vi "四图表串口字符转数字显示.vi"() -> ()   [LabVIEW 2013]
uses:
  <vilib>/Platform/TimedLoop/XDataNode/timing_clust.ctl
  <vilib>/Platform/TimedLoop/XDataNode/nitl_modes.ctl
  <vilib>/Platform/TimedLoop/XDataNode/wakeup.ctl
  <vilib>/Instr/_visa.llb/VISA Configure Serial Port (Instr).vi
  <vilib>/Platform/TimedLoop/XDataNode/XDataNode.xnode
  <vilib>/Platform/TimedLoop/XDataNode/XDNodeRunTimeDep.lvlib
panel:
  out "?":bool
  out "?":bool
  out "?":bool
  in  "预警低温 2":dbl=-5.0
  in  "预警高温 2":dbl=40.0
  out "?":bool
  in  "预警低温":dbl=-5.0
  in  "预警高温":dbl=40.0
  out "光照指示":bool
  in  "关灯时间":timestamp format="%<%H:%M:%S>T"
  in  "?":bool
  in  "?":bool
  out "LED灯":bool
  out "?":dbl
  out "湿度2":u8(graph)
  out "?":dbl
  out "温度2":u8(graph)
  in  "?":bool
  in  "?":bool
  out "?":dbl
  out "?":dbl
  out "红外指示灯":bool
  out "LED灯":bool
  out "湿度1":u8(graph)
  out "温度1":u8(graph)
  out "数值":u32
  in  "开始":bool
  in  "串口号":refnum<visa-resource-name>
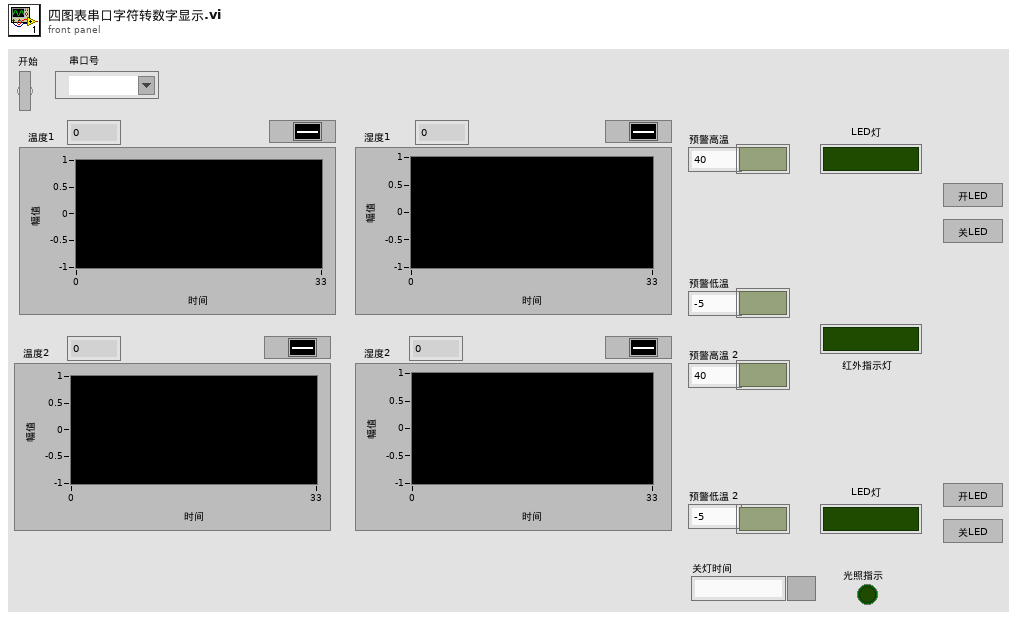
[diagram p1: front panel]
types:
  T1 = typedef "XDNodeRunTimeDep.lvlib/timing_clust.ctl" = cluster{"Expected End [f-1]":u64, "Actual End [f-1]":u64, "Finished Late? [f-1]":bool, "Expected End [i-1]":u64, "Actual End [i-1]":u64, "Finished Late? [i-1]":bool, "Expected Start [i]":u64, "Actual Start [i]":u64, "Expected Start [f]":u64, "Actual Start [f]":u64, "Source Name":string, "Structure Name":string, "Period":i64, "Deadline":i64, "Offset":i64, "Start":i64, "Priority":i32, "Timeout":i32, "Mode":T2, "Wakeup Reason":T3, "Error":errorcluster, "Source Type":string, "Secondary Source Type":string, "Global End Time":u64, "Global Start Time":u64, "Frame Duration":u64, "Iteration Duration":u64, "Assigned CPU":i32, "I/O Scan Engine Mode":u32}
  T2 = typedef "XDNodeRunTimeDep.lvlib/nitl_modes.ctl" = enum32{"No Change", "Process missed periods, maintain original phase", "Discard missed periods, maintain original phase", "Process missed periods, ignore original phase", "Discard missed periods, ignore original phase"}
  T3 = typedef "XDNodeRunTimeDep.lvlib/wakeup.ctl" = enum32{"Normal", "Aborted", "Asynchronous wakeup", "Timing source error", "Timed loop error", "Timeout"}
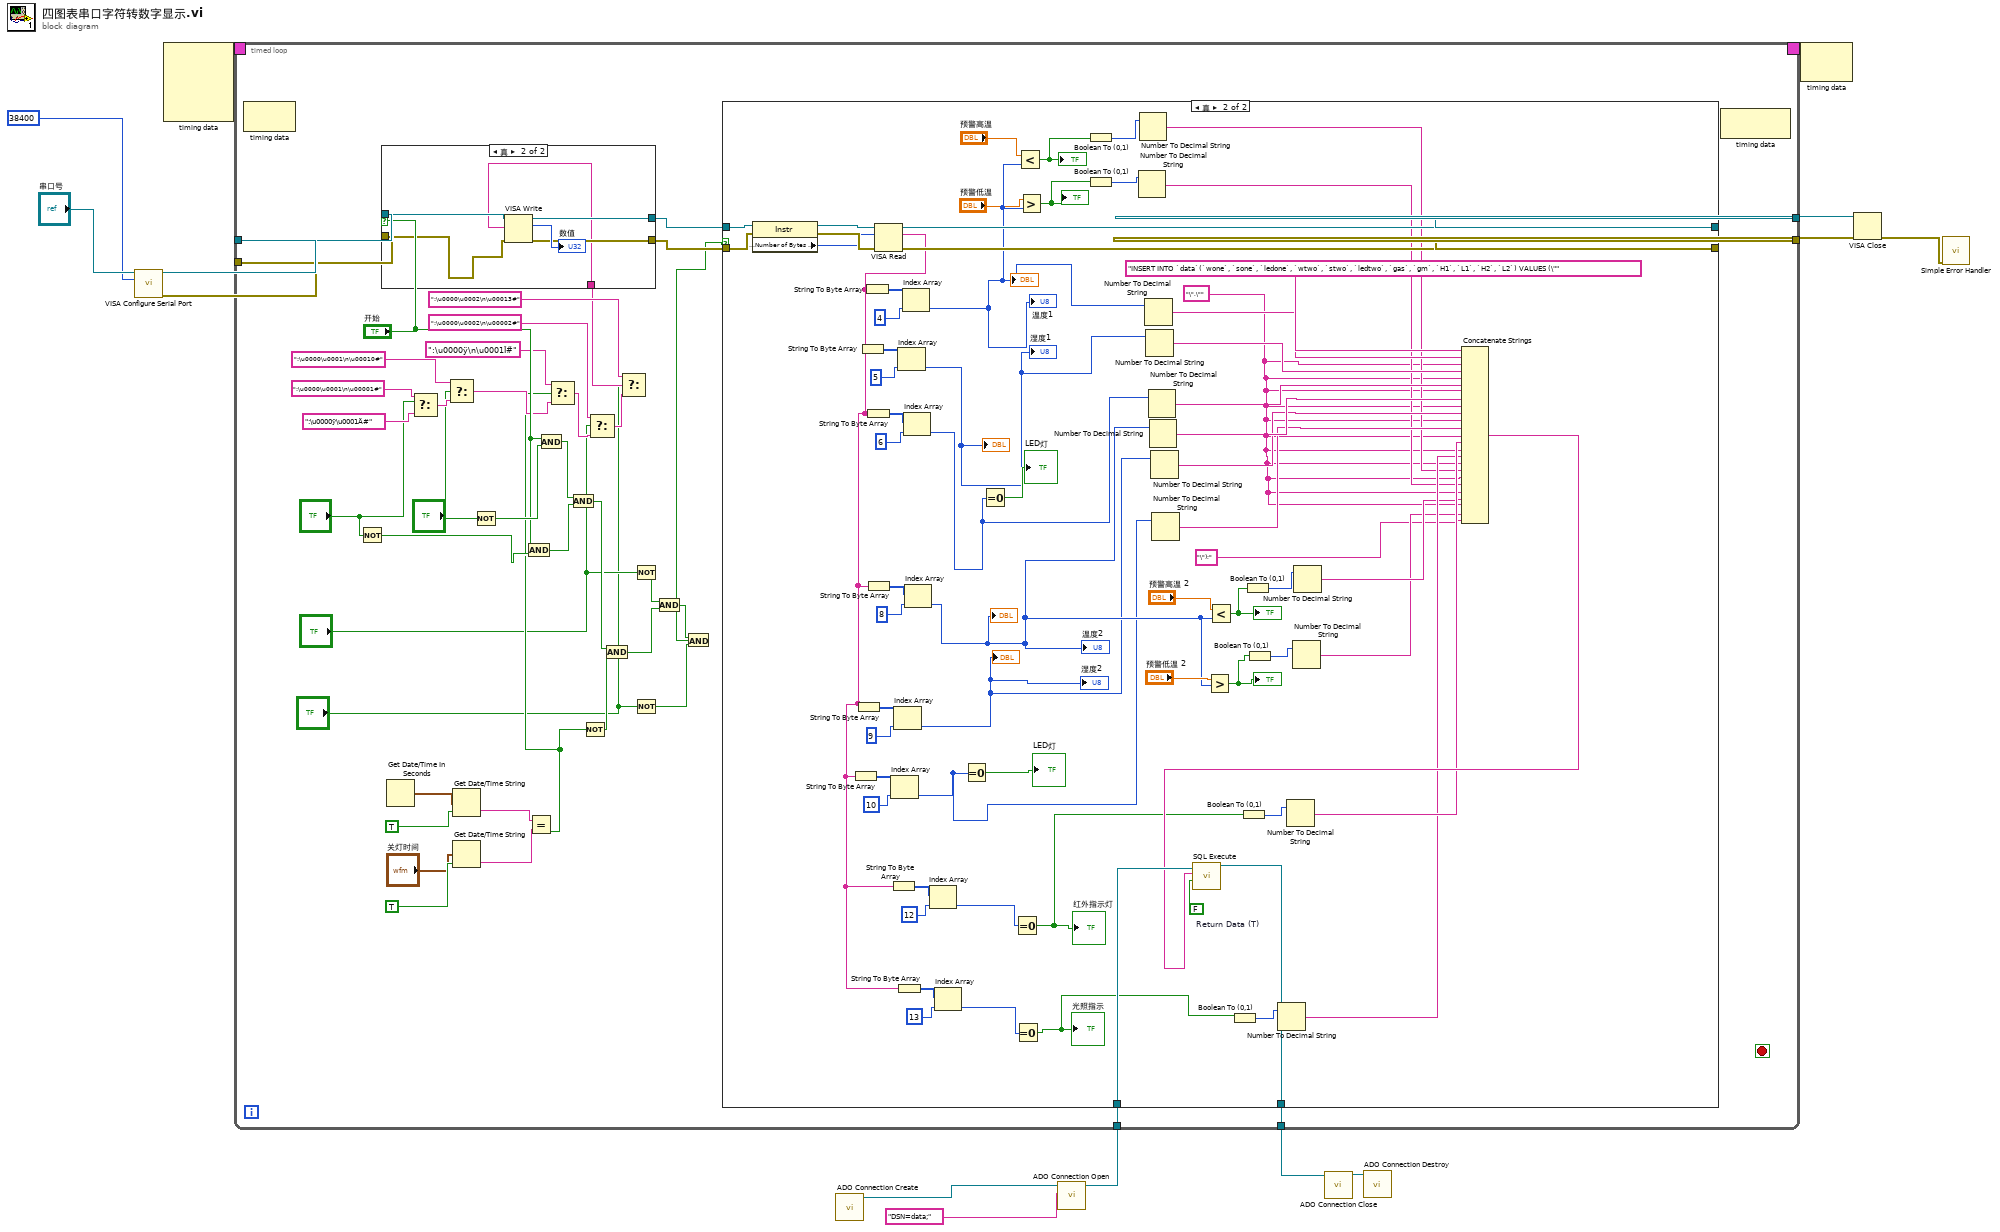
[diagram p0: block diagram]
diagram:
  n1 = call-poly "VISA Configure Serial Port"("VISA resource name"="串口号", "baud rate (9600)"=38400) -> ("VISA resource name out"=w13:refnum<visa-resource-name>, "error out"=w12:errorcluster)  [unwired: 12 in]
  n2 = node-c288() -> (w8:T1)  [unwired: 4 in]
  n3 = call <userlib>:"ADO Connection Create.vi"() -> ("ADODB._Connection Out"=w6:refnum<k7>)  [unwired: 10 in, 1 out]
  n4 = call <userlib>:"ADO Connection Open.vi"("ConnectionString"="DSN=data;", "ADODB._Connection In"=w6) -> ("ADODB._Connection Out"=w4:refnum<k7>)  [unwired: 8 in, 1 out]
  n5 = timed-loop {
    tunnel: w13 -> [w56]
    tunnel: w12 -> [w55]
    tunnel: [w52] -> w11
    tunnel: [w51] -> w10
    timing: w8 -> [_]
    timing-out: [_] -> w7
    tunnel: w4 -> [w29]
    tunnel: [w28] -> w2
    stop <- _ stop-if-true
    n6 = node-c288() -> ()  [unwired: 1 in, 1 out]
    n7 = Not(x="?") -> (.not. x?=w43:bool)
    n8 = Get Date/Time In Seconds ("获取日期/时间（秒）")() -> (seconds since 1Jan1904=w35:timestamp)
    n9 = Select(t=":\u0000\u0001\n\u00001#", s="?", f=":\u0000ÿ\u0001Ä#") -> (s? t:f=w47:string)
    n10 = Select(t=":\u0000\u0001\n\u00010#", s="?", f=w47) -> (s? t:f=w33:string)
    n11 = Get Date/Time String(seconds (now)=w35, want seconds? (F)=TRUE) -> (time string=w36:string)  [unwired: 1 in, 1 out]
    n12 = Get Date/Time String(seconds (now)="关灯时间", want seconds? (F)=TRUE) -> (time string=w38:string)  [unwired: 1 in, 1 out]
    n13 = Not(x="?") -> (.not. x?=w44:bool)
    n14 = And(x="开始", y=w43) -> (x .and. y?=w41:bool)
    n15 = Equal?(x=w36, y=w38) -> (x = y?=w31:bool)
    n16 = And(x="开始", y=w44) -> (x .and. y?=w27:bool)
    n17 = Select(t=":\u0000ÿ\n\u0001Î#", s=w31, f=w33) -> (s? t:f=w26:string)
    n18 = And(x=w27, y=w41) -> (x .and. y?=w34:bool)
    n19 = Not(x=w31) -> (.not. x?=w30:bool)
    n20 = Select(t=":\u0000\u0002\n\u00002#", s="?", f=w26) -> (s? t:f=w24:string)
    n21 = And(x=w34, y=w30) -> (x .and. y?=w18:bool)
    n22 = Select(t=":\u0000\u0002\n\u00013#", s="?", f=w24) -> (s? t:f=w22:string)
    n23 = case shown="真" "开始" {
      tunnel: w56 -> [w131 w137]
      tunnel: w55 -> [w130 w133]
      tunnel: [w131 w135] -> w54
      tunnel: [w130 w134] -> w53
      tunnel: w22 -> [_ w132]
      frame False {
      }
      frame True {
        n24 = VISA Write(VISA resource name=w137, write buffer=w132, error in (no error)=w133) -> (VISA resource name out=w135:refnum<visa-resource-name>, return count=→"数值":u32, error out=w134:errorcluster)
      }
    }
    n25 = Not(x="?") -> (.not. x?=w19:bool)
    n26 = Not(x="?") -> (.not. x?=w16:bool)
    n27 = And(x=w19, y=w18) -> (x .and. y?=w17:bool)
    n28 = And(x=w17, y=w16) -> (x .and. y?=w15:bool)
    n29 = case shown="真" w15 {
      tunnel: w54 -> [w60 w129]
      tunnel: w53 -> [w59 w128]
      tunnel: [w60 w124] -> w52
      tunnel: [w59 w120] -> w51
      tunnel: w29 -> [_ w119]
      tunnel: [_ w118] -> w28
      frame False {
      }
      frame True {
        w121 = FALSE  # Return Data (T)
        w87 = "\",\""
        n30 = property class="Instr"(reference=w129, error in=w128) -> (reference out=w127:refnum<visa-resource-name>, error out=w126:errorcluster, "Serial Settings:Number of Bytes at Serial Port"=w125:u32)
        n31 = VISA Read(VISA resource name=w127, byte count=w125, error in (no error)=w126) -> (VISA resource name out=w124:refnum<visa-resource-name>, read buffer=w61:string, error out=w120:errorcluster)  [unwired: 1 out]
        n32 = String To Byte Array(string=w61) -> (unsigned byte array=w76:u8[])
        n33 = String To Byte Array(string=w61) -> (unsigned byte array=w74:u8[])
        n34 = String To Byte Array(string=w61) -> (unsigned byte array=w82:u8[])
        n35 = String To Byte Array(string=w61) -> (unsigned byte array=w85:u8[])
        n36 = String To Byte Array(string=w61) -> (unsigned byte array=w80:u8[])
        n37 = String To Byte Array(string=w61) -> (unsigned byte array=w78:u8[])
        n38 = String To Byte Array(string=w61) -> (unsigned byte array=w72:u8[])
        n39 = Index Array(array=w76, index=10) -> (element=w64:u8)
        n40 = Index Array(array=w74, index=9) -> (element=w65:u8)
        "湿度2" <- w65
        "?" <- w65
        n41 = String To Byte Array(string=w61) -> (unsigned byte array=w70:u8[])
        n42 = Index Array(array=w82, index=5) -> (element=w68:u8)
        "湿度1" <- w68
        "?" <- w68
        n43 = Index Array(array=w85, index=4) -> (element=w83:u8)
        "温度1" <- w83
        "?" <- w83
        n44 = Index Array(array=w80, index=6) -> (element=w67:u8)
        n45 = Index Array(array=w78, index=8) -> (element=w66:u8)
        "温度2" <- w66
        "?" <- w66
        n46 = Index Array(array=w72, index=12) -> (element=w63:u8)
        n47 = Index Array(array=w70, index=13) -> (element=w62:u8)
        n48 = Equal To 0?(x=w64) -> (x = 0?=→"LED灯":bool)
        n49 = Equal To 0?(x=w67) -> (x = 0?=→"LED灯":bool)
        n50 = Equal To 0?(x=w63) -> (x = 0?=w95:bool)
        "红外指示灯" <- w95
        n51 = Equal To 0?(x=w62) -> (x = 0?=w97:bool)
        "光照指示" <- w97
        n52 = Less?(x="预警高温", y=w83) -> (x < y?=w105:bool)
        "?" <- w105
        n53 = Greater?(x="预警低温", y=w83) -> (0:w104:bool)
        "?" <- w104
        n54 = Boolean To (0,1)(Boolean=w105) -> (0, 1=w99:i16)
        n55 = Boolean To (0,1)(Boolean=w104) -> (0, 1=w98:i16)
        n56 = Number To Decimal String(number=w98) -> (decimal integer string=w90:string)  [unwired: 1 in]
        n57 = Number To Decimal String(number=w99) -> (decimal integer string=w91:string)  [unwired: 1 in]
        n58 = Number To Decimal String(number=w83) -> (decimal integer string=w116:string)  [unwired: 1 in]
        n59 = Number To Decimal String(number=w68) -> (decimal integer string=w115:string)  [unwired: 1 in]
        n60 = Number To Decimal String(number=w67) -> (decimal integer string=w114:string)  [unwired: 1 in]
        n61 = Number To Decimal String(number=w66) -> (decimal integer string=w113:string)  [unwired: 1 in]
        n62 = Number To Decimal String(number=w65) -> (decimal integer string=w112:string)  [unwired: 1 in]
        n63 = Number To Decimal String(number=w64) -> (decimal integer string=w111:string)  [unwired: 1 in]
        n64 = Greater?(x="预警低温 2", y=w66) -> (0:w103:bool)
        "?" <- w103
        n65 = Less?(x="预警高温 2", y=w66) -> (x < y?=w102:bool)
        "?" <- w102
        n66 = Boolean To (0,1)(Boolean=w97) -> (0, 1=w96:i16)
        n67 = Boolean To (0,1)(Boolean=w95) -> (0, 1=w94:i16)
        n68 = Boolean To (0,1)(Boolean=w102) -> (0, 1=w101:i16)
        n69 = Boolean To (0,1)(Boolean=w103) -> (0, 1=w100:i16)
        n70 = Number To Decimal String(number=w96) -> (decimal integer string=w92:string)  [unwired: 1 in]
        n71 = Number To Decimal String(number=w94) -> (decimal integer string=w93:string)  [unwired: 1 in]
        n72 = Number To Decimal String(number=w100) -> (decimal integer string=w88:string)  [unwired: 1 in]
        n73 = Number To Decimal String(number=w101) -> (decimal integer string=w89:string)  [unwired: 1 in]
        n74 = Concatenate Strings("INSERT INTO `data`(`wone`, `sone`, `ledone`, `wtwo`, `stwo`, `ledtwo`, `gas`, `gm`, `H1`, `L1`, `H2`, `L2`) VALUES (\"", w116, w87, w115, w87, w114, w87, w113, w87, w112, w87, w111, w87, w93, w87, w92, w87, w91, w87, w90, w87, w89, w87, w88, "\");") -> (w110:string)
        n75 = call <userlib>:"SQL Execute.vi"("Return Data (T)"=w121, "Command Text"=w110, "ADODB._Connection In"=w119) -> ("ADODB._Connection Out"=w118:refnum<k7>)  [unwired: 5 in, 3 out]
      }
    }
    n76 = node-c288() -> ()  [unwired: 1 in, 1 out]
  }
  n77 = call <userlib>:"ADO Connection Close.vi"("ADODB._Connection In"=w2) -> ("ADODB._Connection Out"=w3:refnum<k7>)  [unwired: 9 in, 1 out]
  n78 = call <userlib>:"ADO Connection Destroy.vi"("ADODB._Connection In"=w3) -> ()  [unwired: 10 in, 1 out]
  n79 = node-c288(w7) -> ()  [unwired: 1 out]
  n80 = VISA Close(VISA resource name=w11, error in (no error)=w10) -> (error out=w9:errorcluster)
  n81 = call <vilib>:"Simple Error Handler.vi"("error in (no error)"=w9) -> ()  [unwired: 4 in, 5 out]
